vi "Get Current Position.vi"(11 "Connection Cluster in":T1) -> (1 "Current position":dbl, 3 "Connection Cluster out":T1, 4 "Response":string)   [LabVIEW 2020]
doc: "TP? - Get Current Position"
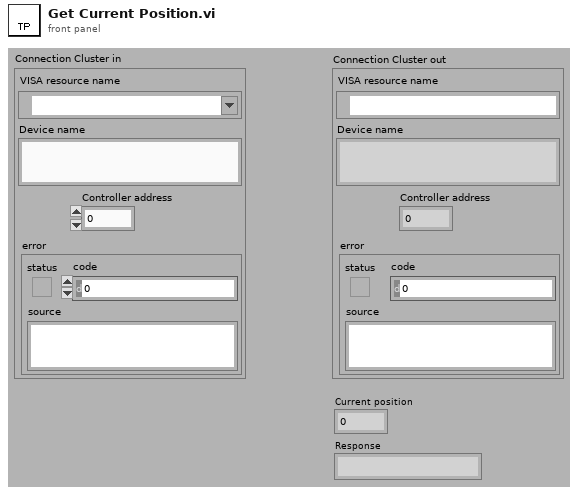
[diagram p1: front panel]
types:
  T1 = cluster{"VISA resource name":refnum<visa-resource-name>, "Device name":string, "Controller address":i32, "error":errorcluster}
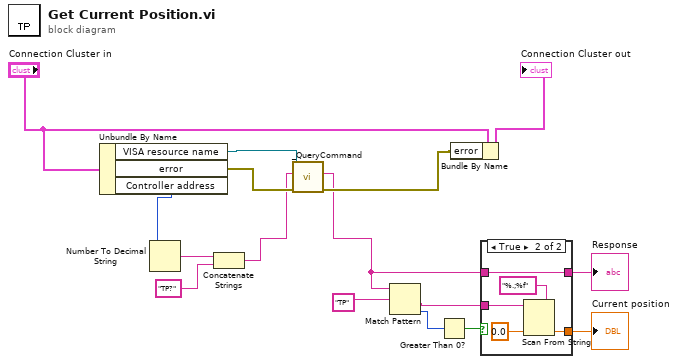
[diagram p0: block diagram]
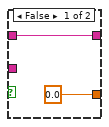
[diagram p2: hidden frame]
diagram:
  n1 = Unbundle By Name("Connection Cluster in") -> ("VISA resource name"=w10:refnum<visa-resource-name>, "error"=w8:errorcluster, "Controller address"=w3:i32)
  n2 = Number To Decimal String(number=w3) -> (decimal integer string=w16:string)  [unwired: 1 out]
  n3 = Concatenate Strings(w16, "TP?" ("strCommand")) -> (w5:string)
  n4 = call "_QueryCommand.vi"("error in"=w8, "Command"=w5, "Instrument Channel in"=w10) -> ("error out"=w9:errorcluster, "Response"=w4:string)  [unwired: 6 in, 1 out]
  n5 = Match Pattern(string=w4, regular expression="TP" ("strCommand")) -> (after substring=w15:string, offset past match=w14:i32)  [unwired: 3 out]
  n6 = Greater Than 0?(x=w14) -> (x > 0?=w13:bool)
  n7 = Bundle By Name(cluster="Connection Cluster in", "error"=w9) -> (→"Connection Cluster out":T1)
  n8 = case shown="True" w13 {
    tunnel: w4 -> [w18 w20]
    tunnel: w15 -> [_ w21]
    tunnel: [w18 w20] -> w12
    tunnel: [0.0 ("valeur par défaut 1") w19] -> w11
    frame False {
    }
    frame True {
      n9 = Scan From String(format string="%.;%f", input string=w21, default 1=0.0 ("valeur par défaut 1")) -> (output 1=w19:dbl)  [unwired: 2 in, 3 out]
    }
  }
  "Response" <- w12
  "Current position" <- w11
